vi "waitForModbus.vi"(8 "error in (no error)":errorcluster, 10 "Timeout (ms)":i32, 11 "FPGA in":refnum<class "FPGA.lvclass">) -> (0 "error out":errorcluster, 2 "Timed Out":bool, 3 "FPGA out":refnum<class "FPGA.lvclass">)   [LabVIEW 2016]
uses:
  FPGA.lvclass
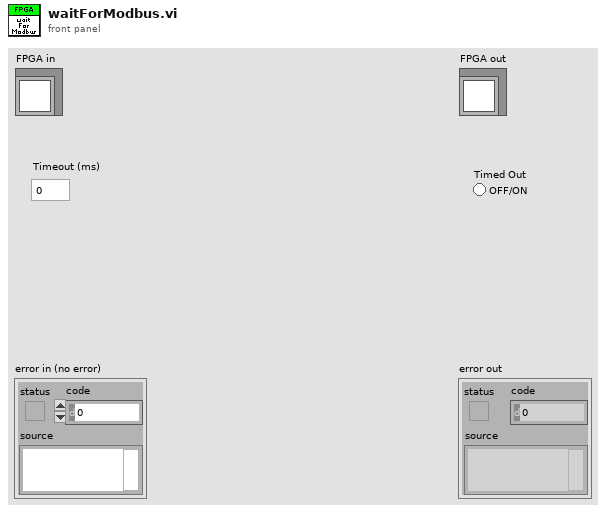
[diagram p1: front panel]
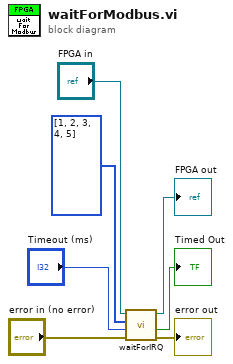
[diagram p0: block diagram]
diagram:
  n1 = call "waitForIRQ.vi"("error in (no error)"="error in (no error)", "Timeout (ms)"="Timeout (ms)", "IRQs in"=i32[] [1, 2, 3, 4, 5], "FPGA in"="FPGA in") -> ("error out"=→"error out":errorcluster, "TimedOut"=→"Timed Out":bool, "FPGA out"=→"FPGA out":refnum<class "FPGA.lvclass">)  [unwired: 4 in, 1 out]
